vi "Fdx Find Resources.vi"(8 "error in":errorcluster, 11 "SrvName (local)":string="local") -> (0 "error out":errorcluster, 2 "Ports":T1[](array[typedef]) {"ServerResourceInfo"."ResourceType" items=["RESOURCETYPE_BOARD"=0, "RESOURCETYPE_PORT"=1, "RESOURCETYPE_ALL"=20]}, 3 "Boards":T2[](array[typedef]) {"ServerResourceInfo"."ResourceType" items=["RESOURCETYPE_BOARD"=0, "RESOURCETYPE_PORT"=1, "RESOURCETYPE_ALL"=20]})   [LabVIEW 2020, in "AIM664LV.lvlib"]
doc: "Query or find all of the resources (boards or ports) in a specific server."
uses:
  AIM664LV.lvlib
  _controls/hwResource_board.ctl
  _controls/hwResource_port.ctl
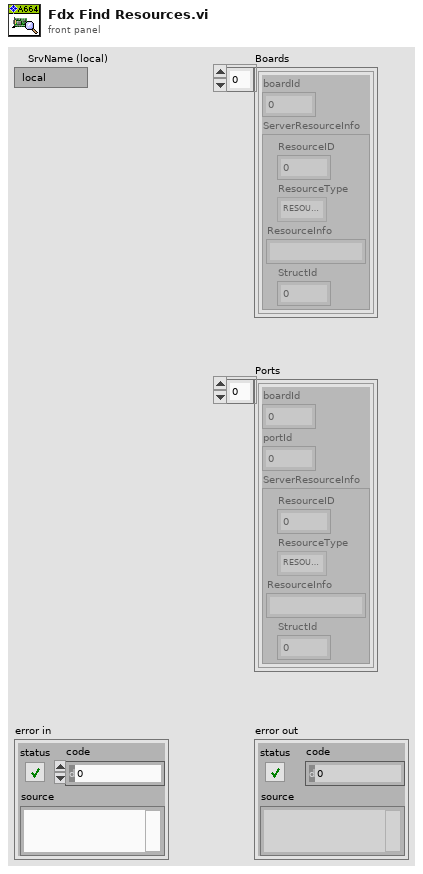
[diagram p1: front panel]
types:
  T1 = typedef "AIM664LV.lvlib/hwResource_port.ctl" = cluster{"boardId":u32, "portId":u32, "ServerResourceInfo":cluster{"ResourceID":u32, "ResourceType":u32, "ResourceInfo":string, "StructId":u32}}
  T2 = typedef "AIM664LV.lvlib/hwResource_board.ctl" = cluster{"boardId":u32, "ServerResourceInfo":cluster{"ResourceID":u32, "ResourceType":u32, "ResourceInfo":string, "StructId":u32}}
  T3 = cluster{"ResourceID":u32, "ResourceType":u32, "ResourceInfo":string, "StructId":u32}
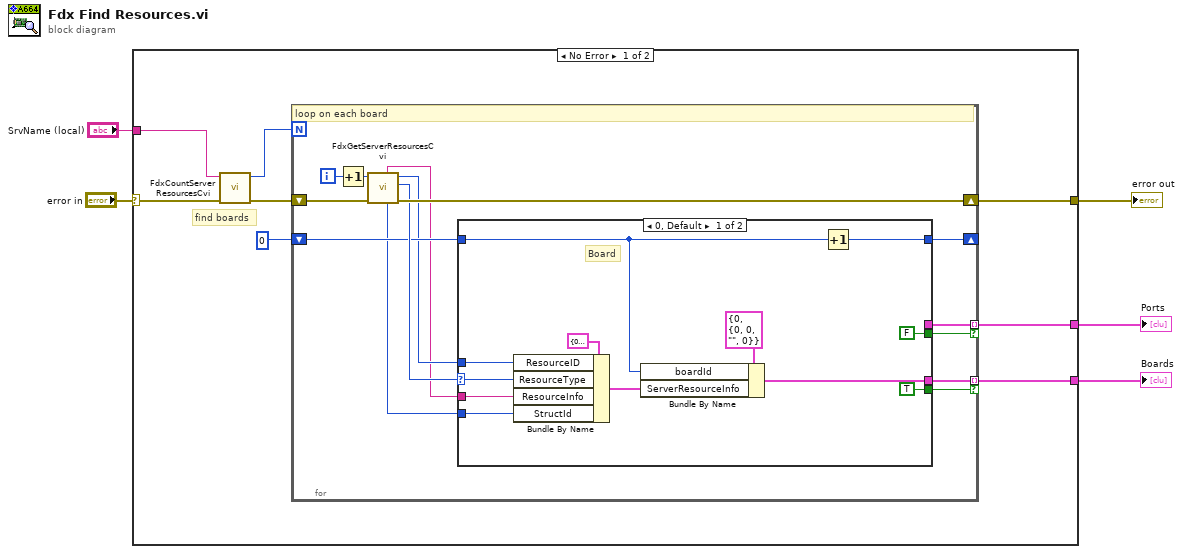
[diagram p0: block diagram]
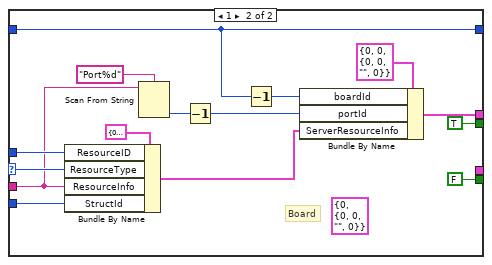
[diagram p2: hidden frame]
diagram:
  n1 = case shown="No Error" "error in" {
    selector: "error in" -> [w7 w55]
    tunnel: [w13 _] -> w5
    tunnel: [w12 _] -> w4
    tunnel: [w6 w55] -> w3
    tunnel: "SrvName (local)" -> [w8 _]
    frame No Error {
      # "find boards"
      n2 = call "FdxCountServerResourcesCvi.vi"("error in"=w7, "SrvName (local)"=w8) -> ("error out"=w9:errorcluster, "Number of Resources"=w10:u32)  [unwired: 8 in]
      n3 = for {
        N: w10 -> [_]
        shift-right: [w25] -> w6
        shift-left: w9 -> [w27]
        shift-right: [w21] -> _
        shift-left: u32 0 -> [w22]
        tunnel: [w20] -> w13 mode=indexing if=w19
        tunnel: [w15] -> w12 mode=indexing if=w14
        i -> [w26]
        # "loop on each board"
        n4 = Increment(x=w26) -> (x+1=w24:i32)
        n5 = call "FdxGetServerResourcesCvi.vi"("error in"=w27, "ServerRElement"=w24) -> ("error out"=w25:errorcluster, "ResourceType"=w23:u32, "Resource ID"=w18:u32, "StructId"=w17:u32, "Resource Info"=w16:string)  [unwired: 4 in, 1 out]
        n6 = case shown="0, Default" w23 {
          selector: w23 -> [w29 w50]
          tunnel: w22 -> [w38 w48]
          tunnel: [w37 w48] -> w21
          tunnel: [w36 _] -> w20
          tunnel: [TRUE FALSE] -> w19
          tunnel: w18 -> [w32 w52]
          tunnel: w17 -> [w31 w51]
          tunnel: w16 -> [w30 w44]
          tunnel: [_ w42] -> w15
          tunnel: [FALSE TRUE] -> w14
          frame 0, Default {
            # "Board"
            n7 = Bundle By Name(cluster=T3 {"ResourceID"=0, "ResourceType"=0, "ResourceInfo"="", "StructId"=0} ("ServerResourceInfo"), "ResourceID"=w32, "ResourceType"=w29, "ResourceInfo"=w30, "StructId"=w31) -> (w33:T3)
            n8 = Bundle By Name(cluster=T2 {"boardId"=0, "ServerResourceInfo"={"ResourceID"=0, "ResourceType"=0, "ResourceInfo"="", "StructId"=0}} ("hw_board"), "boardId"=w38, "ServerResourceInfo"=w33) -> (w36:T2)
            n9 = Increment(x=w38) -> (x+1=w37:u32)
          }
          frame 1 {
            (unwired) T2 {"boardId"=0, "ServerResourceInfo"={"ResourceID"=0, "ResourceType"=0, "ResourceInfo"="", "StructId"=0}} ("hw_board")
            # "Board"
            n10 = Bundle By Name(cluster=T3 {"ResourceID"=0, "ResourceType"=0, "ResourceInfo"="", "StructId"=0} ("ServerResourceInfo"), "ResourceID"=w52, "ResourceType"=w50, "ResourceInfo"=w44, "StructId"=w51) -> (w43:T3)
            n11 = Scan From String(format string="Port%d", input string=w44) -> (output 1=w46:i32)  [unwired: 3 in, 3 out]
            n12 = Decrement(x=w46) -> (x-1=w45:i32)
            n13 = Decrement(x=w48) -> (x-1=w40:u32)
            n14 = Bundle By Name(cluster=T1 {"boardId"=0, "portId"=0, "ServerResourceInfo"={"ResourceID"=0, "ResourceType"=0, "ResourceInfo"="", "StructId"=0}} ("hw_board 2"), "boardId"=w40, "portId"=w45, "ServerResourceInfo"=w43) -> (w42:T1)
          }
        }
      }
    }
    frame Error {
    }
  }
  "Boards" <- w5
  "Ports" <- w4
  "error out" <- w3
